vi "test Deployment No Configuration.vi"(8 "error in":errorcluster, 11 "TestCase in":refnum<class "Deployment.lvclass">) -> (0 "error out":errorcluster, 3 "TestCase out":refnum<class "Deployment.lvclass">)   [LabVIEW 2020, in "Deployment.lvclass"]
uses:
  Deployment.lvclass
  Deployment.lvclass/Deployment.ctl
  315b1c3a-44c8-49e8-b756-01f865c29b4a.vi
  <vilib>/addons/_JKI Toolkits/VI Tester/TestCase.llb/TestCase.lvclass
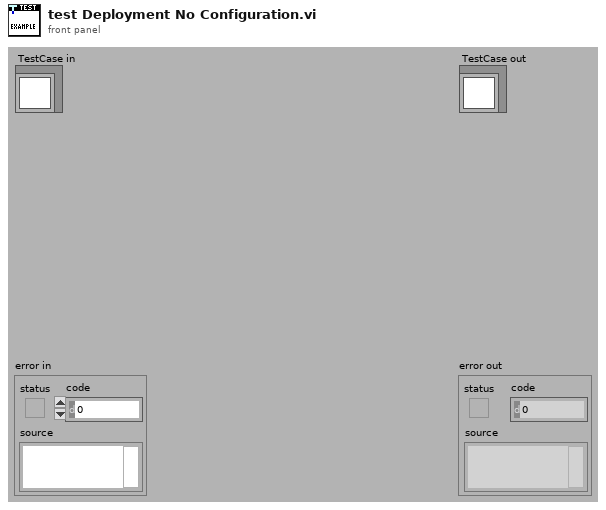
[diagram p1: front panel]
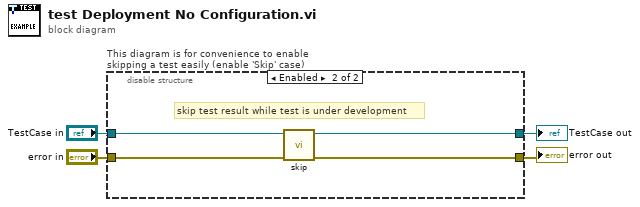
[diagram p0: block diagram]
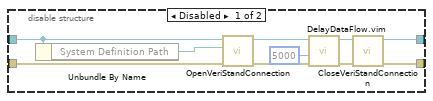
[diagram p2: hidden frame]
diagram:
  n1 = disable-structure "This diagram is for convenience to enable skipping a test easily (enable 'Skip' case)" shown="Enabled" {
    disable-tunnel: "TestCase in" -> [w7 w17]
    disable-tunnel: [w8 w15] -> w1
    disable-tunnel: [w10 w16] -> w3
    disable-tunnel: "error in" -> [w5 w14]
    frame Disabled {
      n2 = Unbundle By Name(w7) -> ("System Definition Path"=w6:path)
      n3 = call-dynamic "OpenVeriStandConnection.vi"("error in (no error)"=w5, "System Definition File"=w6, "VeriStand Test Case in"=w7) -> ("error out"=w13:errorcluster, "VeriStand Test Case out"=w9:refnum<class "Deployment.lvclass">)  [unwired: 6 in, 1 out]
      n4 = call "DelayDataFlow.vim"("value in"=w13, "milliseconds to wait"=u32 5000) -> ("value out"=w11:errorcluster)  [unwired: 2 in, 1 out]
      n5 = call-dynamic "CloseVeriStandConnection.vi"("error in (no error)"=w11, "VeriStand Test Case in"=w9) -> ("error out"=w10:errorcluster, "VeriStand Test Case out"=w8:refnum<class "Deployment.lvclass">)  [unwired: 8 in]
    }
    frame Enabled {
      # "skip test result while test is under development"
      n6 = call <vilib>:"skip.vi"("error in (no error)"=w14, "TestCase in"=w17) -> ("error out"=w16:errorcluster, "TestCase out"=w15:refnum<class "Deployment.lvclass">)  [unwired: 8 in]
    }
  }
  "error out" <- w3
  "TestCase out" <- w1
